vi "Hex String to ASCLL.vi"(11 "Hex String":string="\u0001\u0003až\u0000\u0004:\u001b") -> (3 "ASCII Output":string)   [LabVIEW 2020]
panel:
  # "十进制显示格式的十进制字符串"
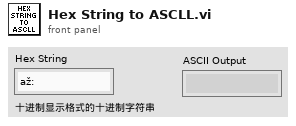
[diagram p1: front panel]
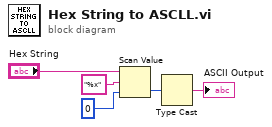
[diagram p0: block diagram]
diagram:
  n1 = Scan Value(string="Hex String", format string="%x", default (0 dbl)=u8 0) -> (value=w2:u8)  [unwired: 1 out]
  n2 = Type Cast(x=w2) -> (*(type *) &x=→"ASCII Output":string)  [unwired: 1 in]
